vi "PoolNoodle.vi"(2 "Joystick":bool[](array[boolean]), 3 "Box":bool[](array[boolean])) -> (0 "Force Pool Noodle":i32, 1 "Force State":i32)   [LabVIEW 2014]
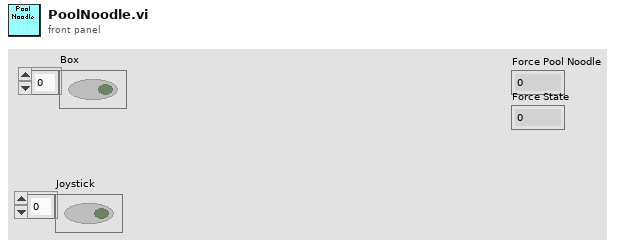
[diagram p1: front panel]
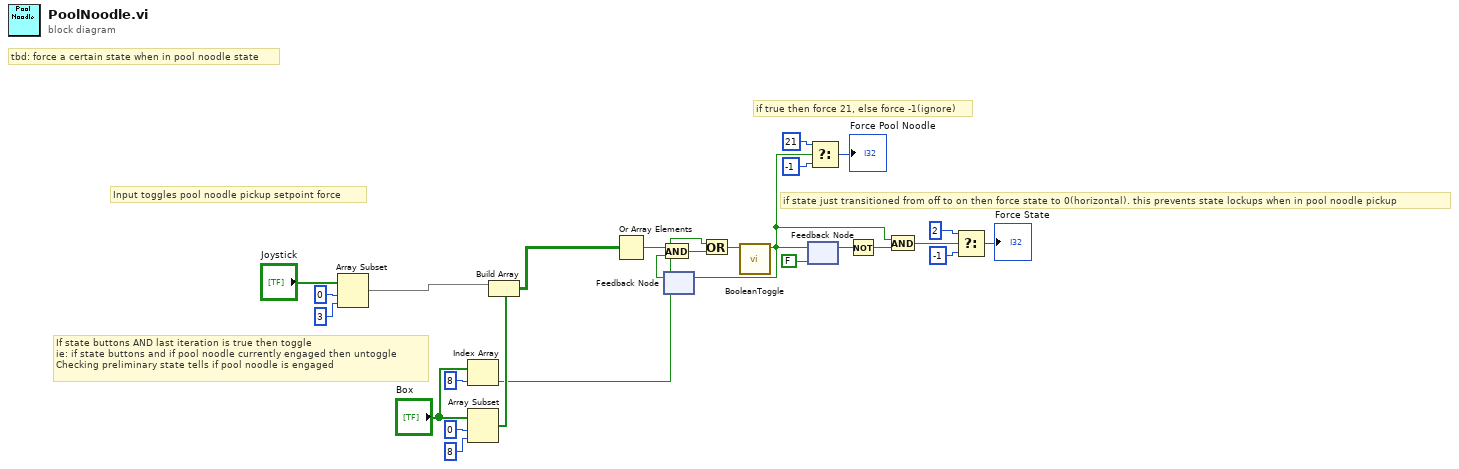
[diagram p0: block diagram]
diagram:
  # "if state just transitioned from off to on then force state to 0(horizontal). this prevents state lockups when in pool noodle pickup"
  # "tbd: force a certain state when in pool noodle state"
  # "if true then force 21, else force -1(ignore)"
  # "If state buttons AND last iteration is true then toggle\nie: if state buttons and if pool noodle currently engaged then untoggle\nChecking preliminary state tells if pool noodle is engaged"
  # "Input toggles pool noodle pickup setpoint force"
  n1 = Array Subset(array="Joystick", index=0, length=3) -> (w1:bool[])
  n2 = Index Array(array="Box", index=8) -> (element=w7:bool)
  n3 = Array Subset(array="Box", index=0, length=8) -> (w9:bool[])
  n4 = Build Array(w1, w9) -> (w6:bool[][])
  n5 = Or Array Elements(Boolean array=w6) -> (logical OR=w22:bool)
  n6 = feedback #1() -> (w23:bool)  [unwired: 1 in]
  n7 = And(x=w22, y=w23) -> (x .and. y?=w20:bool)
  n8 = Or(x=w7, y=w20) -> (x .or. y?=w21:bool)
  n9 = call "BooleanToggle.vi"("Input"=w21) -> ("Output"=w13:bool)  [unwired: 10 in]
  n10 = feedback-in #1(w13) -> ()
  n11 = feedback-in #2(w13) -> ()
  n12 = feedback #2(FALSE ("Output")) -> (w15:bool)
  n13 = Select(t=21, s=w13, f=-1) -> (s? t:f=→"Force Pool Noodle":i32)
  n14 = Not(x=w15) -> (.not. x?=w14:bool)
  n15 = And(x=w13, y=w14) -> (x .and. y?=w12:bool)
  n16 = Select(t=2, s=w12, f=-1) -> (s? t:f=→"Force State":i32)
